vi "Main-Strech DNA-OneDirectionOnly_ver2_YCC.vi"(4 "Avg points":i32=300, 5 "Save Data?":bool, 6 "Who's Data":enum16{"YCC", "PYW", "LCH", "YYH"}(ring), 7 "Set LaserPower (mV)":dbl=-4000.0 format="%0.2f", 8 "File name add to the end \n(laser power-height)":string="FA-h300-1-1", 9 "Record scan rate  (um/s)":dbl=2.0 format="%.3f", 10 "range  (um)":dbl=2.9 format="%.3f", 11 "T=X\nF=Y":bool=TRUE) -> (3 "Stage-QPD Graph":T4(graph))   [LabVIEW 2014]
uses:
  Main-Calibration/WLC fitting/SubVI/WLC-Fitting Cluster.ctl
  <vilib>/Analysis/baseanly.llb/Mean (DBL).vi
  <vilib>/Analysis/NI_AALBase.lvlib
panel:
  out "Axis":i32
  out "Initial Velocity Array":dbl[](array[numeric]) format="%.6f"
  out "center":dbl
  out "avg. Step (nm)":dbl
  in  "WLC fitting?":bool
  in  "Force offset":dbl=800.0
  in  "Length offset":dbl=700.0
  in  "Filter type":T1(ring)=enum."F+S-window avg"
  in  "trap height(nm)":dbl=300.0
  out "Laser Lock?":bool
  in  "xDNA cut outside":dbl=3000.0
  in  "Fitting Cluster 2":T2={"cr (um)"=0.0, "yr (V)"=0.0, "trap height(nm)"=0.0, "bead radius(nm)"=520.0, "Length offset"=0.0, "Upper Force(pN)"=0.0, "cr shift (nm)"=0.0, "yr shift (mV)"=0.0, "LaserPower (mW)"=0.0, "conversion factor (V/um)"=0.0, "Stiffness (pN/nm)"=0.0154, "xDNA cut outside"=0.0, "Lower Force(pN)"=5.0, "c for zbd"=0.0}
  in  "no fec":bool=TRUE
  in  "Avg. time delay (ms)":dbl=18.0
  in  "Use avg delay?":bool=TRUE
  out "delay time between F and U (ms)":dbl
  in  "no Record scan rate  (um/s)":dbl=2.0
  out "Fold QPD Signal (V) 2":dbl[](array[numeric])
  out "Fold Stage Position (um) 2":dbl[](array[numeric])
  out "Folded-Force":dbl[](array[numeric])
  out "Folded-xDNA":dbl[](array[numeric])
  out "Unfolded-Force":dbl[](array[numeric])
  out "Unfolded-xDNA":dbl[](array[numeric])
  out "Filtered QPD Array":dbl[][](array[numeric])
  out "Filtered Stage Array":dbl[][](array[numeric])
  out "Save to File Name Indicator":string
  out "Save to Path Indicator":path
  out "Avg. to Hz":dbl
  out "Fold QPD Signal (V)":dbl[](array[numeric])
  out "Unfold QPD Signal (V)":dbl[](array[numeric])
  out "Fold Stage Position (um)":dbl[](array[numeric])
  out "Unfold Stage Position (um)":dbl[](array[numeric])
  in  "Tab Control":T3(tab)
  out "Stage-QPD Graph 3":T4(graph)
  out "Stage-QPD Graph 2":T4(graph)
  out "Unfolded Graph":cluster{dbl[], dbl[]}(graph)
  out "Folded Graph":cluster{dbl[], dbl[]}(graph)
  out "Unfolded+Folded Graph":T5(graph)
  out "Unfolded Fitting Graph":T6(graph)
  in  "initial parameters for eWLC (Lp,Lc,K)":dbl[](array[numeric])=[45.0, 1800.0, 1200.0]
  in  "initial parameters for marko (Lp,Lc)":dbl[](array[numeric])=[40.0, 1800.0]
  out "best fit parameters\n(Lp,Lc)":dbl[](array[numeric])
  out "best fit parameters\n(Lp,Lc,K)":dbl[](array[numeric])
  out "r^2":dbl
  out "r^2  2":dbl
  in  "eWLC?":bool
  out "Trace direction":bool[](array[boolean])=[FALSE, TRUE, TRUE, FALSE]
  out "Real initial position (um)":dbl format="%0.5f"
  in  "Toward first ?\nT=+, F=-":bool
  in  "Record Mode \npath(1,2)":bool[](array[boolean])=[TRUE, TRUE, FALSE, FALSE]
  in  "Sampling rate":dbl=32000.0 format="%0.2f"
  # "3.8 for full range"
  # "range=3.1um & 4 um/s\n-2000 m¢ä for activead"
  # "avg delay= 33ms\n20181223 ·s¬°18ms"
  # "3281-h300-m51 BRC4 2uM-Ca-ATP-1-8"
  # "3281-h300-sp40-RecA-ATPrS-6"
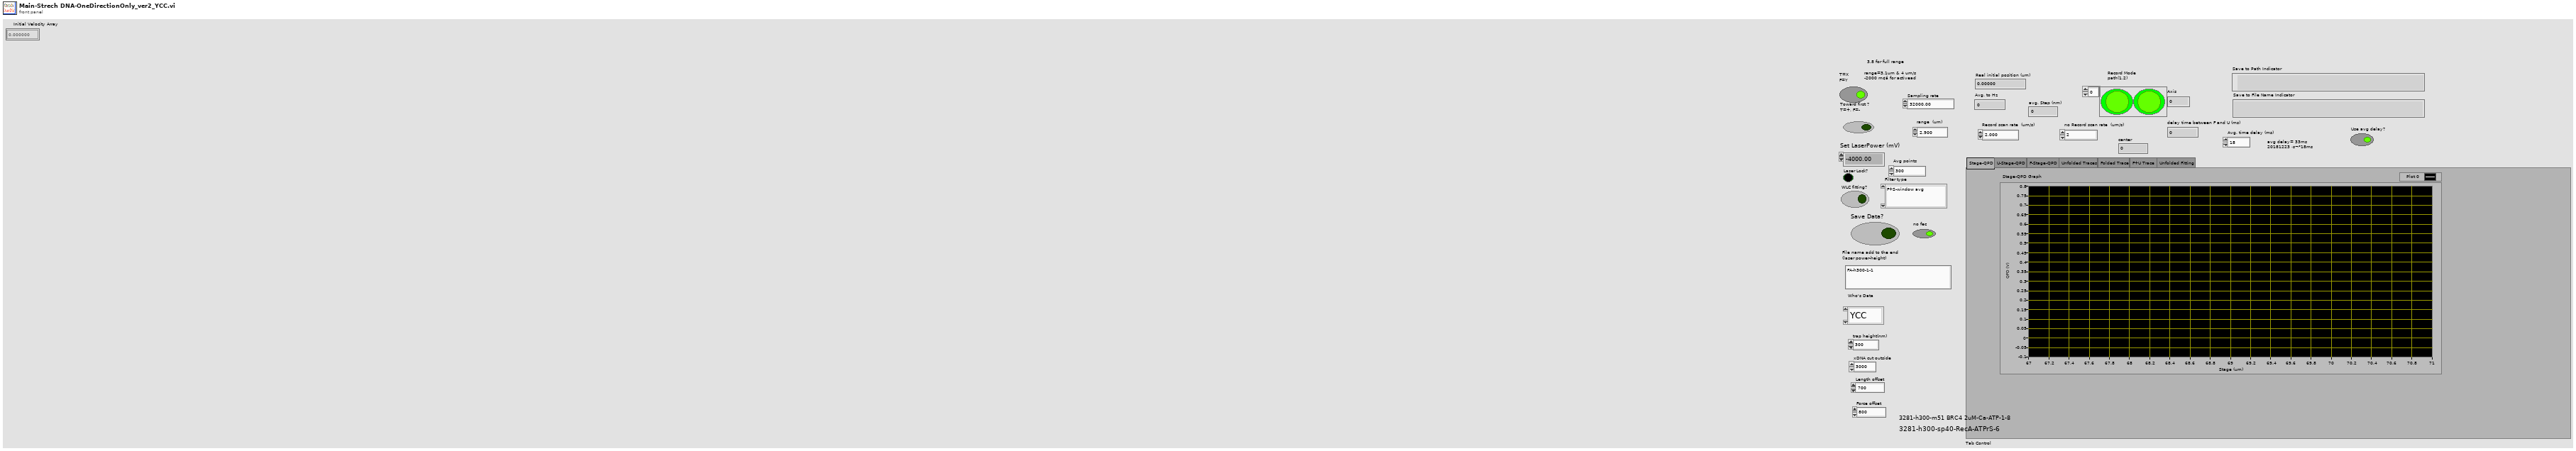
[diagram p1: front panel]
types:
  T1 = enum16{"Fixed-window avg", "Moving-window avg", "F+S-window avg", "S-G filter", "Fixed-window Median", "Moving-window Median "}
  T2 = typedef "WLC-Fitting Cluster.ctl" = cluster{"cr (um)":dbl, "yr (V)":dbl, "trap height(nm)":dbl, "bead radius(nm)":dbl, "Length offset":dbl, "Upper Force(pN)":dbl, "cr shift (nm)":dbl, "yr shift (mV)":dbl, "LaserPower (mW)":dbl, "conversion factor (V/um)":dbl, "Stiffness (pN/nm)":dbl, "xDNA cut outside":dbl, "Lower Force(pN)":dbl, "c for zbd":dbl}
  T3 = enum32{"Stage-QPD", "U-Stage-QPD", "F-Stage-QPD", "Unfolded Traces", "Folded Trace", "F+U Trace", "Unfolded Fitting"}
  T4 = cluster{"Fold Stage Position (um)":dbl[], "Fold QPD Signal (V)":dbl[]}
  T5 = cluster{"Filtered Stage Array":dbl[], "Filtered QPD Array":dbl[]}[]
  T6 = cluster{"best nonlinear fit for Extension (nm)":dbl[], "Force to fit":dbl[]}[]
  T7 = enum16{"Custom", "Centering", "1000 mV", "4500 mV"}
  T8 = cluster{"best nonlinear fit for Extension (nm)":dbl[], "Force to fit":dbl[]}
  T9 = cluster{"Unfolded-xDNA":dbl[], "Unfolded-Force":dbl[]}
  T10 = cluster{"Extension to fit":dbl[], "best nonlinear fit for Force (pN)":dbl[]}
  T11 = cluster{"Folded-xDNA":dbl[], "Folded-Force":dbl[]}
  T12 = cluster{"Folded-xDNA":dbl[], "Folded-Force":dbl[]}[]
  T13 = cluster{"Unfold Stage Position (um)":dbl[], "Unfold QPD Signal (V)":dbl[]}
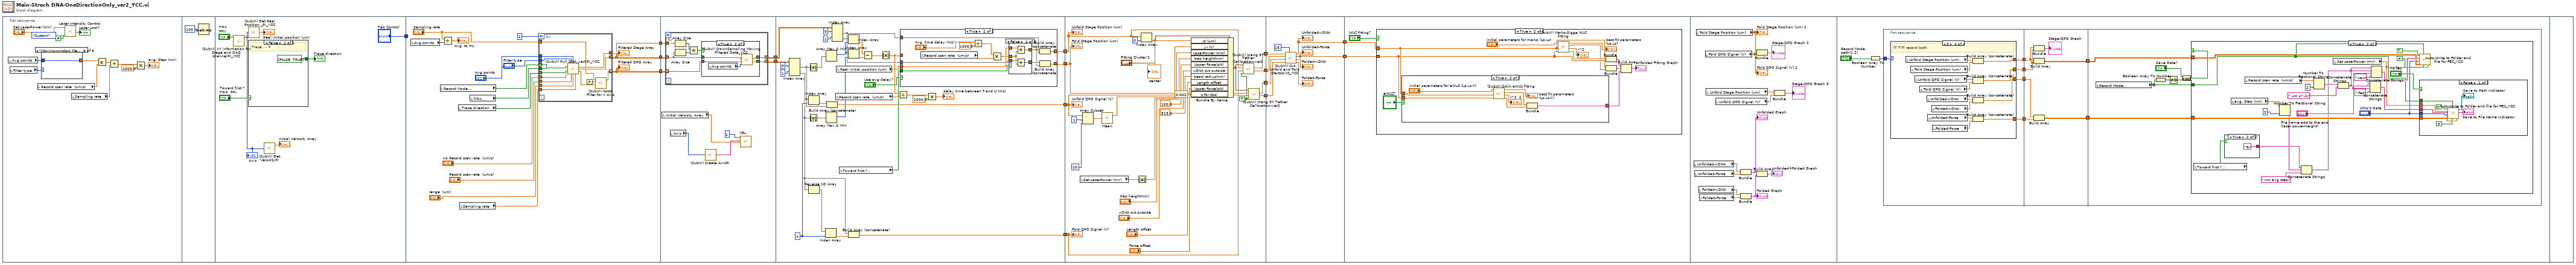
[diagram p0: block diagram]
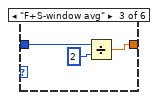
[diagram p4: hidden frame]
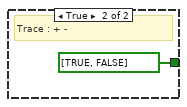
[diagram p7: hidden frame]
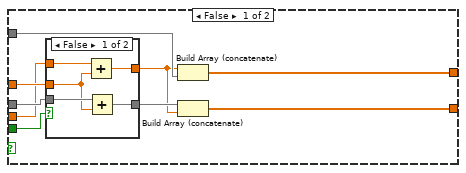
[diagram p9: hidden frame]
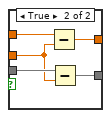
[diagram p10: hidden frame]
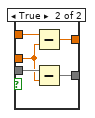
[diagram p11: hidden frame]
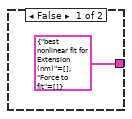
[diagram p13: hidden frame]
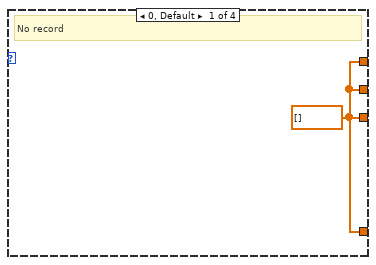
[diagram p14: hidden frame]
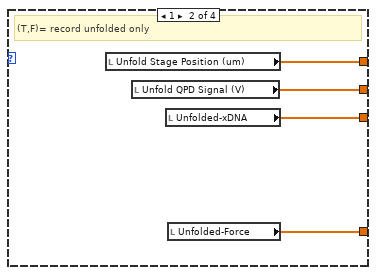
[diagram p15: hidden frame]
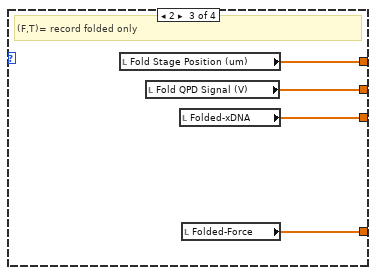
[diagram p16: hidden frame]
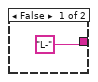
[diagram p18: hidden frame]
diagram:
  n1 = flat-sequence {
    tunnel: ["Tab Control"] -> w16
    tunnel: [w56] -> w5
    tunnel: [w49] -> w7
    tunnel: w16 -> [_]
    tunnel: [w51] -> w3
    tunnel: w7 -> [w86]
    tunnel: [w83] -> w6
    tunnel: w5 -> [w87]
    tunnel: [w84] -> w4
    tunnel: w3 -> [w85]
    tunnel: w6 -> [w130]
    tunnel: w4 -> [w133]
    tunnel: [w115] -> w11
    tunnel: [w110] -> w10
    tunnel: [w109] -> w9
    tunnel: [w112] -> w8
    tunnel: [w201] -> w15
    tunnel: [w200] -> w14
    tunnel: [w199] -> w13
    tunnel: [w198] -> w12
    tunnel: w11 -> [w197]
    tunnel: w10 -> [w186]
    tunnel: w9 -> [w196]
    tunnel: w8 -> [w187]
    tunnel: w15 -> [w212]
    tunnel: w14 -> [w211]
    tunnel: w13 -> [w210]
    tunnel: w12 -> [w208]
    tunnel: [w205] -> w2
    tunnel: [w204] -> w1
    tunnel: w2 -> [w215]
    tunnel: w1 -> [w214]
    frame #0 {
      n2 = local read "Avg points"() -> (w18:i32)
      n3 = local read "Filter type"() -> (w20:T1)
      n4 = local read "Record scan rate  (um/s)"() -> (w26:dbl)
      n5 = case shown="\"Moving-window Median \"" w20 {
        tunnel: [w30 w31 w32 w35 w36 w37] -> w19
        tunnel: w18 -> [w30 w31 w34 w35 w36 w37]
        frame "Fixed-window avg", Default {
        }
        frame "Moving-window avg" {
        }
        frame "F+S-window avg" {
          n6 = Divide(x=w34, y=2) -> (x/y=w32:dbl)
        }
        frame "S-G filter" {
        }
        frame "Fixed-window Median" {
        }
        frame "Moving-window Median " {
        }
      }
      n7 = call "Laser Intensity Control.vi"("Close?"=FALSE, "Enum"=T7."Custom", "Intensity Control, 0~-7000 (mV)"="Set LaserPower (mV)") -> ("Laser Lock?"=→"Laser Lock?":bool)  [unwired: 4 in]
      n8 = local read "Sampling rate"() -> (w24:dbl)
      n9 = Multiply(x=w19, y=w26) -> (x*y=w25:dbl)
      n10 = Divide(x=w25, y=w24) -> (x/y=w23:dbl)
      n11 = Multiply(x=w23, y=1000.0) -> (x*y=→"avg. Step (nm)":dbl)
    }
    frame #1 {
      n12 = Wait (ms)(milliseconds to wait=u32 100) -> ()  [unwired: 1 out]
    }
    frame #2 {
      n13 = call "(SubVI) XY information for Stage and DAQ channelPI_YCC.vi"("T=X\nF=Y"="T=X\nF=Y") -> ("Axis"=w39:i32)  [unwired: 3 in, 1 out]
      "Axis" <- w39
      n14 = call "(SubVI) Get Real Position _PI_YCC.vi"("Axis"=w39) -> ("Real Current Commanded position (um)"=→"Real initial position (um)":dbl)  [unwired: 4 in]
      n15 = case shown="False" "Toward first ?\nT=+, F=-" {
        tunnel: [bool[] [FALSE, TRUE] bool[] [TRUE, FALSE]] -> w42
        frame False {
          # "Trace : - +"
        }
        frame True {
          # "Trace : + -"
        }
      }
      "Trace direction" <- w42
      n16 = call "(SubVI) Get VelocityPI.vi"("axis"=w39) -> ("Velocity Array"=→"Initial Velocity Array":dbl[])  [unwired: 3 in, 1 out]
    }
    frame #3 {
      n17 = local read "Avg points"() -> (w58:i32)
      n18 = local read "Record Mode \npath(1,2)"() -> (w60:bool[])
      n19 = Divide(x="Sampling rate", y=w58) -> (x/y=→"Avg. to Hz":dbl)
      n20 = local read "Trace direction"() -> (w61:bool[])
      n21 = local read "Sampling rate"() -> (w53:dbl)
      n22 = local read "T=X\nF=Y"() -> (w62:bool)
      n23 = for {
        N: 2 -> [_]
        tunnel: "Avg points" -> [w78]
        tunnel: w60 -> [w77] mode=indexing
        tunnel: w62 -> [w76]
        tunnel: w61 -> [w72] mode=indexing
        tunnel: w53 -> [w75]
        tunnel: "Record scan rate  (um/s)" -> [w74]
        tunnel: "range  (um)" -> [w73]
        tunnel: [w69] -> w56 mode=indexing
        tunnel: [w64] -> w49 mode=indexing
        tunnel: "no Record scan rate  (um/s)" -> [w71]
        tunnel: "Filter type" -> [w70]
        tunnel: [w68] -> w51
        tunnel: "Sampling rate" -> [w65]
        n24 = call "(SubVI) Pull DNA_ver2PI_YCC.vi"("Filter type"=w70, "Avg points"=w78, "Record?"=w77, "T=X\nF=Y"=w76, "Toward  ?\nT=+, F=-"=w72, "no Record scan rate  (um/s)"=w71, "Record scan rate  (um/s)"=w74, "range  (um)"=w73, "Sampling rate"=w75) -> ("Raw Stage Array"=w68:dbl[], "Filtered Stage Array"=w69:dbl[], "Filtered QPD Array"=w67:dbl[])  [unwired: 4 in]
        n25 = call "(SubVI) Notch Filter for X Axis.vi"("Sampling rate (Hz)"=w65, "Notch Filter On?"=FALSE, "data"=w67) -> ("Filtered Data"=w64:dbl[])  [unwired: 5 in]
      }
      "Filtered Stage Array" <- w56
      "Filtered QPD Array" <- w49
    }
    frame #4 {
      n26 = local read "Initial Velocity Array"() -> (w80:dbl[])
      n27 = for {
        tunnel: w87 -> [w90] mode=indexing
        tunnel: w86 -> [w92] mode=indexing
        tunnel: w85 -> [w91]
        tunnel: [w89] -> w84 mode=indexing
        tunnel: [w88] -> w83 mode=indexing
        n28 = Array Size(array=w91) -> (size(s)=w93:i32)
        n29 = Array Size(array=w90) -> (size(s)=w94:i32)
        n30 = Equal?(x=w93, y=w94) -> (x = y?=w95:bool)
        n31 = case shown="True" w95 {
          tunnel: w90 -> [w97 w101]
          tunnel: w92 -> [w96 w100]
          tunnel: [w96 w99] -> w88
          tunnel: [w97 w98] -> w89
          frame False {
          }
          frame True {
            n32 = local read "Avg points"() -> (w102:i32)
            n33 = call "(SubVI) DownSampling Moving Filtered Data_YCC.vi"("data# reduce factor"=w102, "Moving Filtered QPD data"=w100, "Moving Filtered Stage data"=w101) -> ("DownSampling QPD"=w99:dbl[], "DownSampling Stage"=w98:dbl[])  [unwired: 3 in]
          }
        }
      }
      n34 = local read "Axis"() -> (w79:i32)
      n35 = call "(SubVI) Create AxisPI.vi"("axis"=w79) -> ("Axis String Array"=w81:string[])  [unwired: 2 in, 2 out]
      n36 = call "VEL.vi"("System no."=1, "Axes to set"=w81, "Velocity values"=w80) -> ()  [unwired: 3 in, 14 out]
    }
    frame #5 {
      w107 = 4 ("index")
      n37 = Index Array(array=w130, index (row) #1=0 ("index (row)"), index (row) #2=1 ("index (row)")) -> (element #1=w108:dbl[], element #2=w104:dbl[])  [unwired: 2 in]
      n38 = Absolute Value(x=w108) -> (abs(x)=w129:dbl[])
      n39 = Absolute Value(x=w104) -> (abs(x)=w128:dbl[])
      n40 = Index Array(array=w108, index=w107) -> (element=w106:dbl)
      n41 = Reverse 1D Array(array=w104) -> (reversed array=w103:dbl[])
      n42 = Index Array(array=w103, index=w107) -> (element=w105:dbl)
      n43 = Array Max & Min(array=w129) -> (max index (indices)=w125:i32)  [unwired: 3 out]
      n44 = Array Max & Min(array=w128) -> (max index (indices)=w124:i32)  [unwired: 3 out]
      n45 = Build Array (concatenate)(w106, w108) -> (w110:dbl[])
      n46 = Index Array(array=w133, index (row) #1=0 ("index (row)"), index (row) #2=1 ("index (row)")) -> (element #1=w113:dbl[], element #2=w117:dbl[])  [unwired: 2 in]
      n47 = local read "Record scan rate  (um/s)"() -> (w119:dbl)
      n48 = local read "Real initial position (um)"() -> (w111:dbl)
      n49 = local read "Toward first ?\nT=+, F=-"() -> (w118:bool)
      n50 = Index Array(array=w113, index=w125) -> (element=w127:dbl)
      n51 = Index Array(array=w117, index=w124) -> (element=w126:dbl)
      n52 = Build Array (concatenate)(w104, w105) -> (w109:dbl[])
      n53 = Subtract(x=w127, y=w126) -> (x-y=w120:dbl)
      n54 = Absolute Value(x=w120) -> (abs(x)=w116:dbl)
      n55 = Divide(x=w116, y=w119) -> (x/y=w123:dbl)
      n56 = case shown="True" "Use avg delay?" {
        tunnel: w118 -> [w144 w165]
        tunnel: w117 -> [w143 w166]
        tunnel: w116 -> [w142 _]
        tunnel: [w137 w156] -> w115
        tunnel: w113 -> [w141 w160]
        tunnel: [w140 w159] -> w112
        tunnel: w111 -> [w136 w155]
        frame False {
          n57 = case shown="False" w144 {
            tunnel: w143 -> [w149 w154]
            tunnel: w142 -> [w146 w151]
            tunnel: [w148 w153] -> w139
            tunnel: w136 -> [w147 w152]
            tunnel: [w145 w150] -> w138
            frame False {
              n58 = Add(x=w147, y=w146) -> (x+y=w145:dbl)
              n59 = Add(x=w149, y=w146) -> (x+y=w148:dbl[])
            }
            frame True {
              n60 = Subtract(x=w152, y=w151) -> (x-y=w150:dbl)
              n61 = Subtract(x=w154, y=w151) -> (x-y=w153:dbl[])
            }
          }
          n62 = Build Array (concatenate)(w138, w141) -> (w140:dbl[])
          n63 = Build Array (concatenate)(w139, w138) -> (w137:dbl[])
        }
        frame True {
          n64 = local read "Record scan rate  (um/s)"() -> (w167:dbl)
          n65 = Divide(x="Avg. time delay (ms)", y=1000.0) -> (x/y=w162:dbl)
          n66 = Multiply(x=w162, y=w167) -> (x*y=w164:dbl)
          n67 = case shown="False" w165 {
            tunnel: w166 -> [w172 w177]
            tunnel: w164 -> [w169 w174]
            tunnel: [w171 w176] -> w158
            tunnel: w155 -> [w170 w175]
            tunnel: [w168 w173] -> w157
            frame False {
              n68 = Add(x=w170, y=w169) -> (x+y=w168:dbl)
              n69 = Add(x=w172, y=w169) -> (x+y=w171:dbl[])
            }
            frame True {
              n70 = Subtract(x=w175, y=w174) -> (x-y=w173:dbl)
              n71 = Subtract(x=w177, y=w174) -> (x-y=w176:dbl[])
            }
          }
          n72 = Build Array (concatenate)(w157, w160) -> (w159:dbl[])
          n73 = Build Array (concatenate)(w158, w157) -> (w156:dbl[])
        }
      }
      n74 = Multiply(x=w123, y=1000.0) -> (x*y=→"delay time between F and U (ms)":dbl)
    }
    frame #6 {
      w179 = TRUE ("X=T\nY=F")
      n75 = local read "Set LaserPower (mV)"() -> (w191:dbl)
      n76 = Array Subset(array=w186, index=1, length=10) -> (w183:dbl[])
      n77 = call-poly <vilib>:"Mean.vi"("X"=w183) -> ("mean"=w182:dbl)  [unwired: 1 out]
      n78 = Absolute Value(x=w191) -> (abs(x)=w190:dbl)
      n79 = Index Array(array=w187, index=0) -> (element=w202:dbl)
      "center" <- w202
      n80 = Bundle By Name(cluster="Fitting Cluster 2", "cr (um)"=w202, "yr (V)"=w182, "LaserPower (mW)"=w190, "trap height(nm)"="trap height(nm)", "Upper Force(pN)"=100.0 ("Force offset"), "xDNA cut outside"="xDNA cut outside", "bead radius(nm)"=515.0, "Length offset"="Length offset", "Upper Force(pN)"="Force offset", "c for zbd"=0.002) -> (w194:T2)
      n81 = call "(SubVI) Wang 97 Tether Calibration-ver2.vi"("X=T\nY=F"=w179, "QPD signal"=w186, "Stage Position"=w187, "Fitting Cluster"=w194) -> ("Force"=w200:dbl[], "xDNA"=w201:dbl[])  [unwired: 1 in, 1 out]
      n82 = call "(SubVI) Wang 97 Tether Calibration-ver2.vi"("X=T\nY=F"=w179, "QPD signal"=w196, "Stage Position"=w197, "Fitting Cluster"=w194) -> ("Force"=w198:dbl[], "xDNA"=w199:dbl[])  [unwired: 1 in, 1 out]
      "Unfold Stage Position (um)" <- w187
      "Fold Stage Position (um)" <- w197
      "Unfold QPD Signal (V)" <- w186
      "Fold QPD Signal (V)" <- w196
    }
    frame #7 {
      n83 = call "(SubVI) Cut Unfold and Fold Startpoint_YCC.vi"("number to cut"=15, "Folded-Force in"=w208, "Folded-xDNA in"=w210, "Unfolded-Force"=w211, "Unfolded-xDNA"=w212) -> ("Folded-Force"=→"Folded-Force":dbl[], "Folded-xDNA"=→"Folded-xDNA":dbl[], "Unfolded-Force"=w204:dbl[], "Unfolded-xDNA"=w205:dbl[])  [unwired: 3 in]
      "Unfolded-Force" <- w204
      "Unfolded-xDNA" <- w205
    }
    frame #8 {
      n84 = case shown="True" "WLC fitting?" {
        tunnel: w215 -> [_ w224]
        tunnel: w214 -> [_ w223]
        frame False {
        }
        frame True {
          n85 = case shown="True" "eWLC?" {
            tunnel: w224 -> [_ w233]
            tunnel: w223 -> [_ w232]
            tunnel: [T8 {"best nonlinear fit for Extension (nm)"=[], "Force to fit"=[]} w229] -> w218
            frame False {
            }
            frame True {
              n86 = call "(SubVI) Odijk eWLC fitting.vi"("Force (pN)"=w232, "Extension (nm)"=w233, "initial parameters for eWLC (Lp,Lc,K=1200)"="initial parameters for eWLC (Lp,Lc,K)") -> ("Force to fit"=w230:dbl[], "r^2"=→"r^2  2":dbl, "best nonlinear fit for Extension (nm)"=w231:dbl[], "best fit parameters\n(Lp,Lc,K=1200)"=→"best fit parameters\n(Lp,Lc,K)":dbl[])  [unwired: 1 in]
              n87 = Bundle("best nonlinear fit for Extension (nm)"=w231, "Force to fit"=w230) -> (w229:T8)  [unwired: 1 in]
            }
          }
          n88 = call "(SubVI) Marko-Sigga WLC fitting.vi"("Force (pN)"=w223, "Extension (nm)"=w224, "initial parameters for marko"="initial parameters for marko (Lp,Lc)") -> ("Extension to fit"=w222:dbl[], "r^2"=→"r^2":dbl, "best nonlinear fit for Force (pN)"=w221:dbl[], "best fit parameters\n(Lp,Lc)"=→"best fit parameters\n(Lp,Lc)":dbl[])  [unwired: 1 in]
          n89 = Bundle("Unfolded-xDNA"=w224, "Unfolded-Force"=w223) -> (w220:T9)  [unwired: 1 in]
          n90 = Bundle("Extension to fit"=w222, "best nonlinear fit for Force (pN)"=w221) -> (w219:T10)  [unwired: 1 in]
          n91 = Build Array(w220, w219, w218) -> (→"Unfolded Fitting Graph":T6)
        }
      }
    }
    frame #9 {
      n92 = local read "Unfolded-xDNA"() -> (w249:dbl[])
      n93 = local read "Unfolded-Force"() -> (w248:dbl[])
      n94 = local read "Fold Stage Position (um)"() -> (w241:dbl[])
      "Fold Stage Position (um) 2" <- w241
      n95 = local read "Folded-xDNA"() -> (w246:dbl[])
      n96 = local read "Folded-Force"() -> (w245:dbl[])
      n97 = local read "Fold QPD Signal (V)"() -> (w240:dbl[])
      "Fold QPD Signal (V) 2" <- w240
      n98 = local read "Unfold Stage Position (um)"() -> (w239:dbl[])
      n99 = local read "Unfold QPD Signal (V)"() -> (w238:dbl[])
      n100 = Bundle("Unfolded-xDNA"=w249, "Unfolded-Force"=w248) -> (w247:T9)  [unwired: 1 in]
      "Unfolded Graph" <- w247
      n101 = Bundle("Folded-xDNA"=w246, "Folded-Force"=w245) -> (w243:T11)  [unwired: 1 in]
      "Folded Graph" <- w243
      n102 = Bundle("Fold Stage Position (um)"=w241, "Fold QPD Signal (V)"=w240) -> (→"Stage-QPD Graph 2":T4)  [unwired: 1 in]
      n103 = Build Array(w247, w243) -> (→"Unfolded+Folded Graph":T12)
      n104 = Bundle("Unfold Stage Position (um)"=w239, "Unfold QPD Signal (V)"=w238) -> (→"Stage-QPD Graph 3":T13)  [unwired: 1 in]
    }
    frame #10 {
      n105 = Boolean Array To Number(Boolean array="Record Mode \npath(1,2)") -> (number=w256:u32)
      n106 = flat-sequence {
        tunnel: w256 -> [w260]
        tunnel: [w262] -> w255
        tunnel: [w261] -> w254
        tunnel: [w259] -> w252
        tunnel: [w258] -> w251
        tunnel: w255 -> [w286]
        tunnel: w254 -> [w285]
        tunnel: [w290] -> w253
        tunnel: w252 -> [w289]
        tunnel: w251 -> [w288]
        tunnel: [w287] -> w250
        tunnel: w253 -> [w294]
        tunnel: w250 -> [w291]
        frame #0 {
          n107 = case shown="3" w260 {
            tunnel: [w263 w267 w271 w279] -> w262
            tunnel: [w263 w266 w270 w278] -> w261
            tunnel: [w263 w265 w269 w273] -> w259
            tunnel: [w263 w264 w268 w272] -> w258
            frame 0, Default {
              w263 = dbl[] [] ("Fold Stage Position (um)")
              # "No record"
            }
            frame 1 {
              # "(T,F)= record unfolded only"
              n108 = local read "Unfold Stage Position (um)"() -> (w267:dbl[])
              n109 = local read "Unfold QPD Signal (V)"() -> (w266:dbl[])
              n110 = local read "Unfolded-xDNA"() -> (w265:dbl[])
              n111 = local read "Unfolded-Force"() -> (w264:dbl[])
            }
            frame 2 {
              # "(F,T)= record folded only"
              n112 = local read "Fold Stage Position (um)"() -> (w271:dbl[])
              n113 = local read "Fold QPD Signal (V)"() -> (w270:dbl[])
              n114 = local read "Folded-xDNA"() -> (w269:dbl[])
              n115 = local read "Folded-Force"() -> (w268:dbl[])
            }
            frame 3 {
              # "(T,T)= record both"
              n116 = local read "Unfold Stage Position (um)"() -> (w283:dbl[])
              n117 = local read "Fold Stage Position (um)"() -> (w282:dbl[])
              n118 = local read "Unfold QPD Signal (V)"() -> (w281:dbl[])
              n119 = local read "Fold QPD Signal (V)"() -> (w280:dbl[])
              n120 = local read "Unfolded-xDNA"() -> (w277:dbl[])
              n121 = local read "Unfolded-Force"() -> (w275:dbl[])
              n122 = local read "Folded-xDNA"() -> (w276:dbl[])
              n123 = local read "Folded-Force"() -> (w274:dbl[])
              n124 = Build Array (concatenate)(w283, w282) -> (w279:dbl[])
              n125 = Build Array (concatenate)(w281, w280) -> (w278:dbl[])
              n126 = Build Array (concatenate)(w277, w276) -> (w273:dbl[])
              n127 = Build Array (concatenate)(w275, w274) -> (w272:dbl[])
            }
          }
        }
        frame #1 {
          n128 = Bundle("Fold Stage Position (um)"=w286, "Fold QPD Signal (V)"=w285) -> (→"Stage-QPD Graph":T4)  [unwired: 1 in]
          n129 = Build Array(w286, w285) -> (w290:dbl[][])
          n130 = Build Array(w289, w288) -> (w287:dbl[][])
        }
        frame #2 {
          n131 = local read "Record Mode \npath(1,2)"() -> (w292:bool[])
          n132 = Boolean Array To Number(Boolean array=w292) -> (number=w293:u32)
          n133 = Not Equal To 0?(x=w293) -> (x != 0?=w296:bool)
          n134 = And(x="Save Data?", y=w296) -> (x .and. y?=w295:bool)
          n135 = case shown="True" w295 {
            tunnel: w294 -> [_ w314]
            tunnel: w292 -> [_ w316]
            tunnel: w291 -> [_ w315]
            frame False {
            }
            frame True {
              n136 = local read "Toward first ?\nT=+, F=-"() -> (w299:bool)
              n137 = case shown="True" w299 {
                tunnel: ["L-" "R-"] -> w298
                frame False {
                }
                frame True {
                }
              }
              n138 = local read "avg. Step (nm)"() -> (w304:dbl)
              n139 = local read "Record scan rate  (um/s)"() -> (w310:dbl)
              n140 = Number To Fractional String(number=w304, precision (6)=i16 2) -> (F-format string=w302:string)  [unwired: 2 in]
              n141 = Concatenate Strings(w298, w302, " nm avg step-") -> (w300:string)
              n142 = Number To Fractional String(number=w310, precision (6)=i16 2) -> (F-format string=w311:string)  [unwired: 2 in]
              n143 = local read "Set LaserPower (mV)"() -> (w306:dbl)
              n144 = Concatenate Strings(w311, " um s^-1-") -> (w305:string)
              n145 = Concatenate Strings(w305, w300, "File name add to the end \n(laser power-height)", "-fec" ("string")) -> (w320:string)
              n146 = Concatenate Strings(w305, w300, "File name add to the end \n(laser power-height)", "-raw" ("string")) -> (w317:string)
              n147 = call "Auto-Write to Folder and file for FEC_YCC.vi"("Current PD (mV)"=w306, "Centering data?"=FALSE, "Record Mode \npath(1,2)"=w316, "data to be saved"=w314, "Who's Data"="Who's Data", "File name add to the end \n(height)"=w317, "Save?"=TRUE) -> ()  [unwired: 1 in, 2 out]
              n148 = case shown="False" "no fec" {
                tunnel: w320 -> [w330 _]
                tunnel: w316 -> [w329 _]
                tunnel: w315 -> [w328 _]
                tunnel: "Who's Data" -> [w326 _]
                tunnel: w306 -> [w325 _]
                frame False {
                  n149 = call "Auto-Write to Folder and file for FEC_YCC.vi"("Current PD (mV)"=w325, "Centering data?"=FALSE, "Record Mode \npath(1,2)"=w329, "data to be saved"=w328, "Who's Data"=w326, "File name add to the end \n(height)"=w330, "Save?"=TRUE) -> ("Save to File Name"=→"Save to File Name Indicator":string, "Save to Path"=→"Save to Path Indicator":path)  [unwired: 1 in]
                }
                frame True {
                }
              }
            }
          }
        }
      }
    }
    frame #11 {
    }
  }
